vi "配置握手.vi"(8 "error in (no error)":errorcluster caption="错误输入（无错误）", 11 "串口 输入":refnum<class "串口.lvclass"> caption="DNL_LabVIEW Object in") -> (0 "error out":errorcluster caption="错误输出", 3 "串口 输出":refnum<class "串口.lvclass"> caption="DNL_LabVIEW Object out")   [LabVIEW 2012, in "串口.lvclass"]
panel:
  in  "Handshaking":i32(ring) items=["None", "XOnXOff", "RequestToSend", "RequestToSendXOnXOff"]
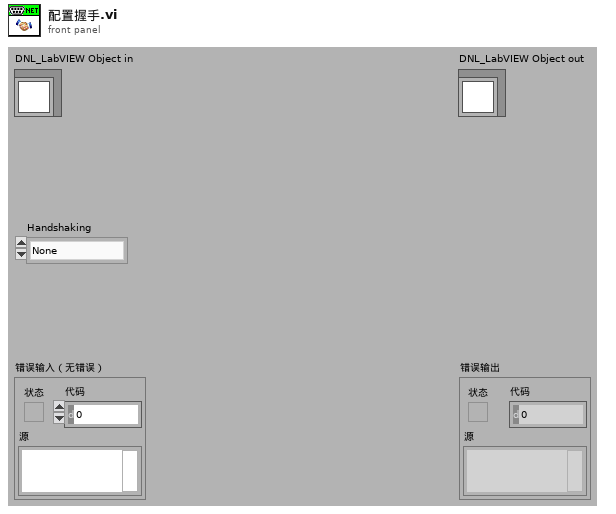
[diagram p1: front panel]
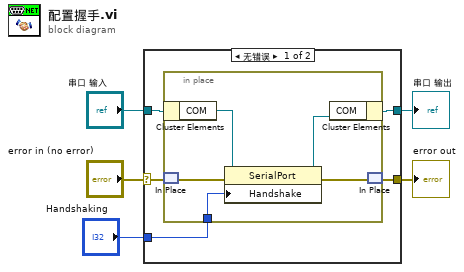
[diagram p0: block diagram]
diagram:
  n1 = case shown="无错误" "error in (no error)" {
    selector: "error in (no error)" -> [w7 w17]
    tunnel: [w6 w17] -> w4
    tunnel: [w9 w16] -> w2
    tunnel: "串口 输入" -> [w10 w16]
    tunnel: "Handshaking" -> [w8 _]
    frame No Error {
      n2 = in-place {
        in-place-border: w8 -> [w13]
        n3 = in-place-cluster #1(w10) -> ("COM"=w15:refnum<k24>)
        n4 = in-place-match #2(w7) -> (w12:errorcluster)
        n5 = property class="SerialPort"(reference=w15, error in=w12, "Handshake"=w13) -> (reference out=w14:refnum<k24>, error out=w11:errorcluster)
        n6 = in-place-cluster #1("COM"=w14) -> (w9:refnum<class "串口.lvclass">)
        n7 = in-place-match #2(w11) -> (w6:errorcluster)
      }
    }
    frame Error {
    }
  }
  "error out" <- w4
  "串口 输出" <- w2
